vi "Batch-Import-User-Channels GUID Lookup.vi"() -> ()   [LabVIEW 2015, in "Batch-Import-User-Channels Custom Device.lvlib"]
doc: "Use this Global VI to access the GUIDs assigned to the page resources of the Custom Device."
uses:
  Batch-Import-User-Channels Custom Device.lvlib
panel:
  in  "Custom Device":string="a54dc6fa-9b45-4bcc-a197-52abfde7fb89"
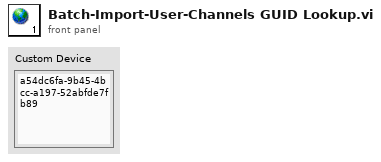
[diagram p1: front panel]
diagram:
